vi "Generate Control Command.vi"(6 "Maximum Speed":u8 max=100, 8 "Error In":errorcluster, 9 "Motor On":bool, 10 "Steering wheel":i8 min=-100 max=100, 11 "Speed":i8 min=-100 max=100) -> (0 "Error Out":errorcluster, 2 "Servo Command":string, 3 "Motor Command":string)   [LabVIEW 2014]
doc: "This VI generates command from input data."
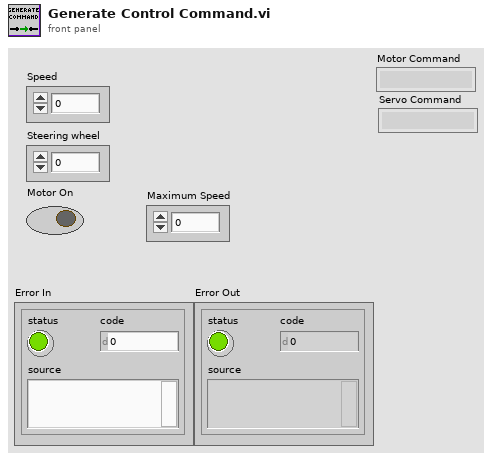
[diagram p1: front panel]
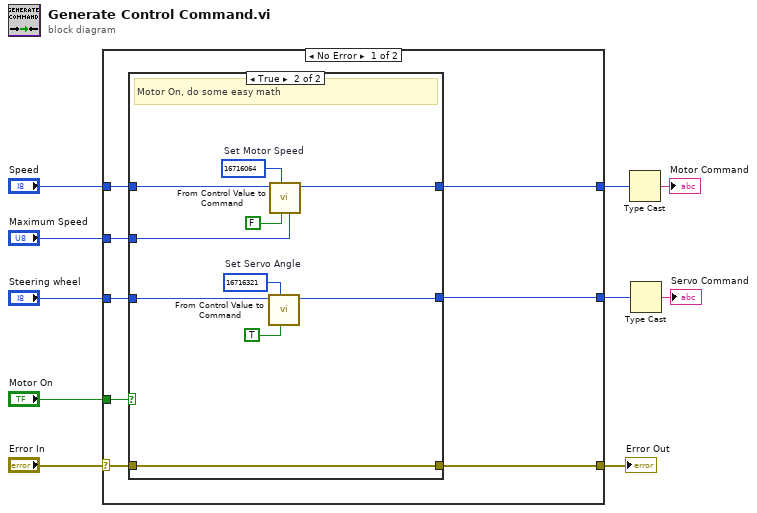
[diagram p0: block diagram]
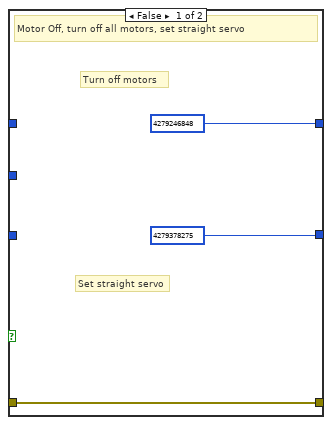
[diagram p2: hidden frame]
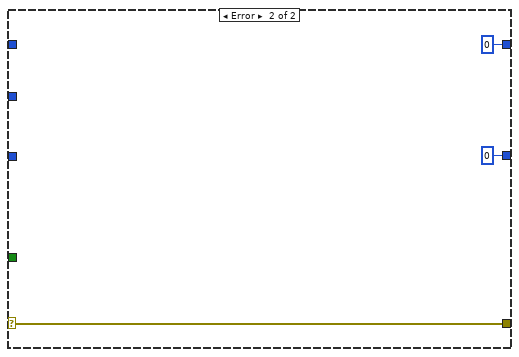
[diagram p3: hidden frame]
diagram:
  n1 = case shown="No Error" "Error In" {
    selector: "Error In" -> [w13 w34]
    tunnel: [w12 w34] -> w9
    tunnel: "Motor On" -> [w18 _]
    tunnel: "Steering wheel" -> [w15 _]
    tunnel: "Speed" -> [w14 _]
    tunnel: [w17 u32 0 ("Command in Hex")] -> w4
    tunnel: [w16 u32 0 ("Command in Hex")] -> w5
    tunnel: "Maximum Speed" -> [w11 _]
    frame No Error {
      n2 = case shown="True" w18 {
        tunnel: [u32 4279378275 w25] -> w17
        tunnel: [u32 4279246848 w28] -> w16
        tunnel: w15 -> [_ w27]
        tunnel: w14 -> [_ w30]
        tunnel: w13 -> [w19 w31]
        tunnel: [w19 w31] -> w12
        tunnel: w11 -> [_ w22]
        frame False {
          # "Set straight servo"
          # "Turn off motors"
          # "Motor Off, turn off all motors, set straight servo"
        }
        frame True {
          w26 = u32 16716321  # Set Servo Angle
          w29 = u32 16716064  # Set Motor Speed
          # "Motor On, do some easy math"
          n3 = call "From Control Value to Command.vi"("Servo?"=TRUE, "Command Beginning"=w26, "From -100 to 100"=w27) -> ("Command in Hex"=w25:u32)  [unwired: 7 in, 1 out]
          n4 = call "From Control Value to Command.vi"("Maximum Speed"=w22, "Servo?"=FALSE, "Command Beginning"=w29, "From -100 to 100"=w30) -> ("Command in Hex"=w28:u32)  [unwired: 6 in, 1 out]
        }
      }
    }
    frame Error {
    }
  }
  "Error Out" <- w9
  n5 = Type Cast(x=w5) -> (*(type *) &x=→"Motor Command":string)  [unwired: 1 in]
  n6 = Type Cast(x=w4) -> (*(type *) &x=→"Servo Command":string)  [unwired: 1 in]
